vi "AppleScript Main.vi"(11 "Mode":i32) -> ()   [LabVIEW 2015]
doc: "Main block for AppleScript.\nPut this in the autonomous vi. Do not place this inside of a loop."
uses:
  <vilib>/Rock Robotics/Network Tables/NT Read String.vi
panel:
  # "AppleScript\nAutonomous Scripting Language for LabVIEW\nCreated by Cory Lynch\nFRC Team 2067"
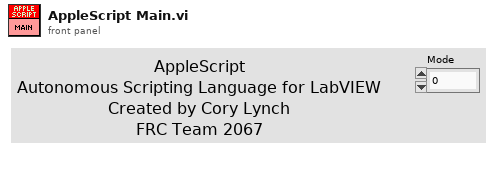
[diagram p1: front panel]
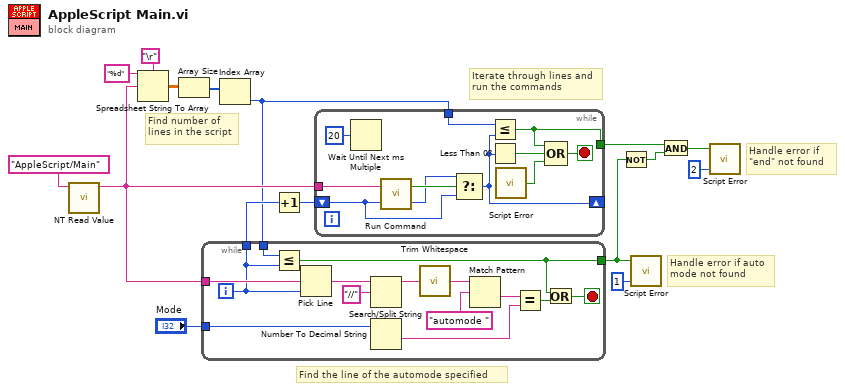
[diagram p0: block diagram]
diagram:
  # "Find number of \nlines in the script"
  # "Handle error if\n\"end\" not found"
  # "Handle error if auto\nmode not found"
  # "Iterate through lines and\nrun the commands"
  # "Find the line of the automode specified"
  n1 = call-poly <vilib>:"NT Read Value.vi"("Name"="AppleScript/Main") -> ("String"=w10:string)  [unwired: 9 in, 1 out]
  n2 = Spreadsheet String To Array(delimiter (Tab)="\r", format string="%d", spreadsheet string=w10) -> (array=w14:dbl[][])  [unwired: 1 in]
  n3 = Array Size(array=w14) -> (size(s)=w11:i32[])
  n4 = Index Array(array=w11) -> (element=w4:i32)  [unwired: 1 in]
  n5 = while {
    tunnel: w10 -> [w23]
    tunnel: "Mode" -> [w29]
    tunnel: [w19] -> w16
    tunnel: w4 -> [w20]
    tunnel: [w17] -> w3
    i -> [w19]
    stop <- w18 stop-if-true
    n6 = Less Or Equal?(x=w20, y=w19) -> (x <= y?=w17:bool)
    n7 = Pick Line(multi-line string=w23, line index=w19) -> (output string=w22:string)  [unwired: 1 in]
    n8 = Search/Split String(string=w22, search string/char (-)="//") -> (substring before match=w25:string)  [unwired: 1 in, 2 out]
    n9 = Number To Decimal String(number=w29) -> (decimal integer string=w27:string)  [unwired: 1 in]
    n10 = call <vilib>:"Trim Whitespace.vi"("string"=w25) -> ("trimmed string"=w24:string)  [unwired: 1 in]
    n11 = Match Pattern(string=w24, regular expression="automode ") -> (after substring=w28:string)  [unwired: 1 in, 3 out]
    n12 = Equal?(x=w28, y=w27) -> (x = y?=w21:bool)
    n13 = Or(x=w17, y=w21) -> (x .or. y?=w18:bool)
  }
  n14 = Increment(x=w16) -> (x+1=w2:i32)
  n15 = while {
    tunnel: w10 -> [w41]
    shift-right: [w38] -> _
    shift-left: w2 -> [w40]
    tunnel: w4 -> [w37]
    tunnel: [w36] -> w7
    stop <- w34 stop-if-true
    n16 = Wait Until Next ms Multiple(millisecond multiple=u32 20 ("milliseconds to wait")) -> ()  [unwired: 1 out]
    n17 = call "Run Command.vi"("Line Index In"=w40, "Script"=w41) -> ("Line Index Out"=w31:i32, "Done"=w39:bool)
    n18 = Select(t=w31, s=w39, f=w40) -> (s? t:f=w38:i32)
    n19 = Less Or Equal?(x=w37, y=w38) -> (x <= y?=w36:bool)
    n20 = Less Than 0?(x=w38) -> (x < 0?=w35:bool)
    n21 = call "Script Error.vi"() -> ("Error?"=w33:bool)  [unwired: 5 in]
    n22 = Compound Arithmetic op=OR(w36, w35, w33) -> (w34:bool)
  }
  n23 = Not(x=w3) -> (.not. x?=w6:bool)
  n24 = call "Script Error.vi"("Error?"=w3, "Error Code"=1) -> ()  [unwired: 3 in, 1 out]
  n25 = And(x=w7, y=w6) -> (x .and. y?=w5:bool)
  n26 = call "Script Error.vi"("Error?"=w5, "Error Code"=2) -> ()  [unwired: 3 in, 1 out]
